vi "TEMPLATE_Regular_NoReturn.vi"(8 "Error In":errorcluster, 11 "QObject In":refnum<class "QObject.lvclass">) -> (0 "Error Out":errorcluster, 3 "QObject Out":refnum<class "QObject.lvclass">)   [LabVIEW 2013, in "Template.lvlib" / "QObject.lvclass"]
uses:
  QObject.lvclass
  QObject.lvclass/QObject.ctl
  LQWidgetEngine/LQWidgetEngine.lvclass
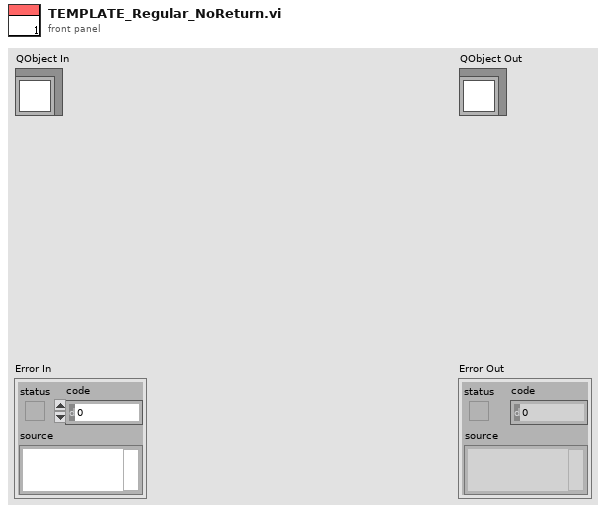
[diagram p1: front panel]
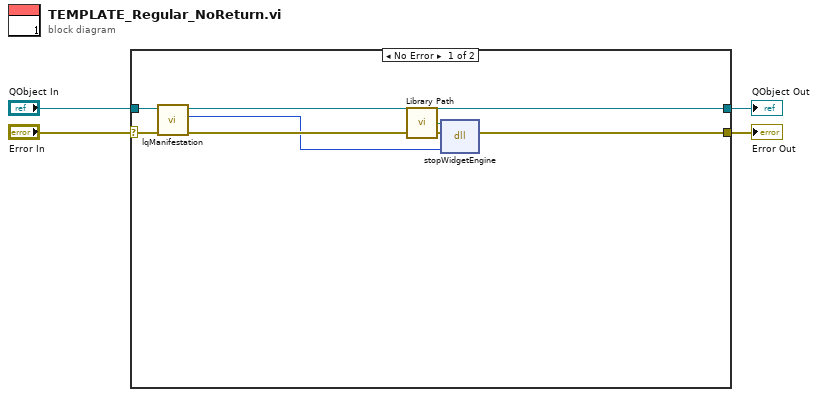
[diagram p0: block diagram]
diagram:
  n1 = case shown="No Error" "Error In" {
    selector: "Error In" -> [w8 w13]
    tunnel: [w11 w13] -> w3
    tunnel: [w9 w12] -> w1
    tunnel: "QObject In" -> [w10 w12]
    frame No Error {
      n2 = call "lqManifestation.vi"("error in (no error)"=w8, "QObject in"=w10) -> ("error out"=w7:errorcluster, "Manifestation"=w5:u32, "QObject out"=w9:refnum<class "QObject.lvclass">)  [unwired: 7 in]
      n3 = call "Library Path.vi"() -> ("Library Path"=w6:path)
      n4 = dll-call lib="?" fn="stopWidgetEngine"(path in=w6, error in=w7, "obj"=w5) -> (error out=w11:errorcluster)  [unwired: 3 in, 1 out]
    }
    frame Error {
    }
  }
  "Error Out" <- w3
  "QObject Out" <- w1
